vi "Flat_Secuence.vi"() -> ()   [LabVIEW 2020]
panel:
  out "Thermometer 3":u16(slide) scale=0.0..100.0
  out "Thermometer 2":u16(slide) scale=0.0..100.0
  out "Thermometer":u16(slide) scale=0.0..100.0
  # "Flat Secuence"
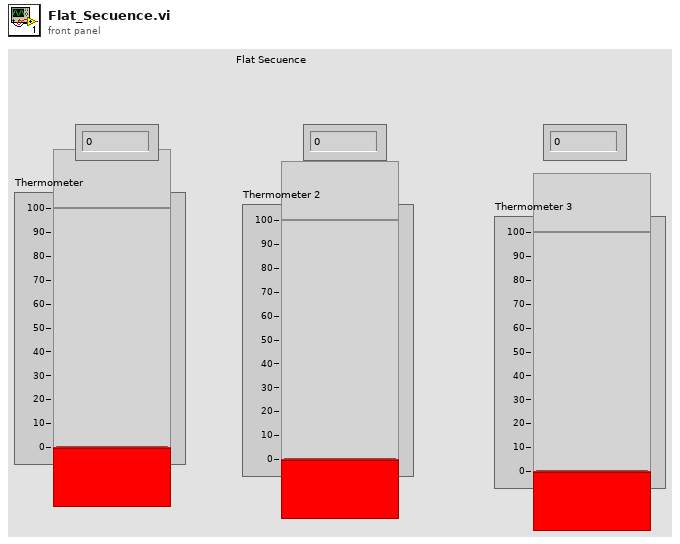
[diagram p1: front panel]
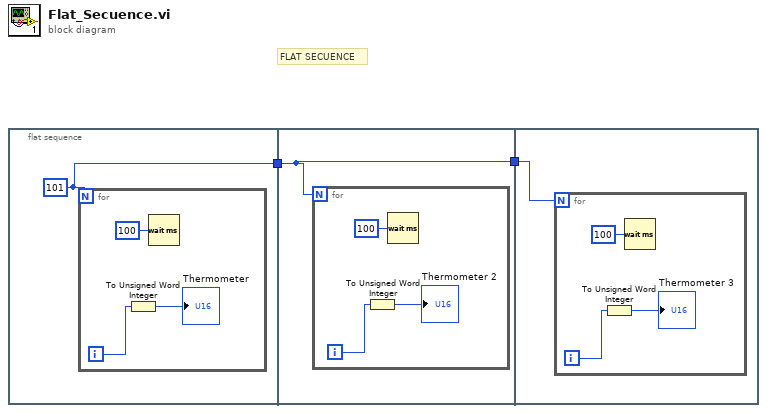
[diagram p0: block diagram]
diagram:
  # "FLAT SECUENCE"
  n1 = flat-sequence {
    tunnel: [w3] -> w2
    tunnel: w2 -> [w7]
    tunnel: [w7] -> w1
    tunnel: w1 -> [w11]
    frame #0 {
      w3 = 101
      n2 = for {
        N: w3 -> [_]
        i -> [w5]
        n3 = To Unsigned Word Integer(number=w5) -> (unsigned 16bit integer=→"Thermometer":u16)
        n4 = Wait (ms)(milliseconds to wait=u32 100) -> ()  [unwired: 1 out]
      }
    }
    frame #1 {
      n5 = for {
        N: w7 -> [_]
        i -> [w9]
        n6 = To Unsigned Word Integer(number=w9) -> (unsigned 16bit integer=→"Thermometer 2":u16)
        n7 = Wait (ms)(milliseconds to wait=u32 100) -> ()  [unwired: 1 out]
      }
    }
    frame #2 {
      n8 = for {
        N: w11 -> [_]
        i -> [w13]
        n9 = To Unsigned Word Integer(number=w13) -> (unsigned 16bit integer=→"Thermometer 3":u16)
        n10 = Wait (ms)(milliseconds to wait=u32 100) -> ()  [unwired: 1 out]
      }
    }
  }
